vi "Get Connection Settings.vi"(11 "Model in":refnum<class "Model.lvclass">) -> (2 "Connection Settings":T1={"Pressure Servo Valve 1 DAC"=1, "Pressure Servo Valve 2 DAC"=2, "Turbo Valve DAC"=3, "Load Cell ADC"=1, "FC1 ILC Port"="", "FC2 ILC Port"="", "Tovey A-B Port"="", "Tovey C-F Port"="", "Tovey D-E Port"="", "FC1 ILC Protocol"=enum."RS485", "FC2 ILC Protocol"=enum."RS485", "Tovey A-B Protocol"=enum."RS485", "Tovey C-F Protocol"=enum."RS485", "Tovey D-E Protocol"=enum."RS485", "Tovey A-B Address"=3, "Tovey C-F Address"=1, "Tovey D-E Address"=1, "Bias DAC"=4, "Axial Push Channel"="ai0", "Axial Pull Channel"="ai1", "Lateral Push Channel"="ai2", "Lateral Pull Channel"="ai3", "TV Control"="ao0", "TV Bias"="ao1", "Rate"=200} {"Rate" min=1; "Bias DAC" min=1 max=4; "Tovey D-E Address" min=1; "Tovey C-F Address" min=1; "Tovey A-B Address" min=1; "Load Cell ADC" min=1 max=4; "Turbo Valve DAC" min=1 max=4; "Pressure Servo Valve 2 DAC" min=1 max=4; "Pressure Servo Valve 1 DAC" min=1 max=4}, 3 "Model out":refnum<class "Model.lvclass">)   [LabVIEW 2015, in "Model.lvclass"]
uses:
  Model.lvclass
  Typedefs/Connection Settings.ctl
  <userlib>/Common/SerialProtocols/Configuration/SerialProtocol.ctl
  Model.lvclass/Model.ctl
  <userlib>/Common/SerialProtocols/SerialProtocols.lvlib
  Typedefs/FAMT Typedefs.lvlib
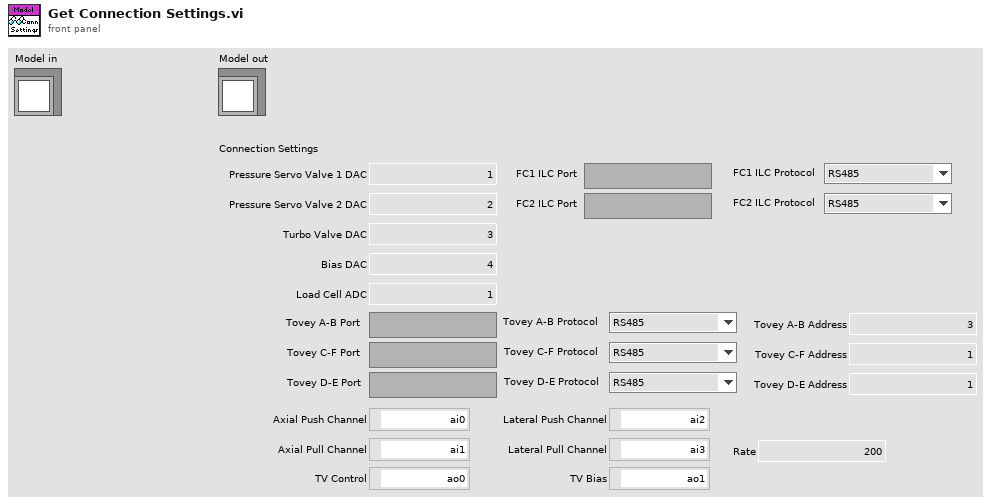
[diagram p1: front panel]
types:
  T1 = typedef "FAMT Typedefs.lvlib/Connection Settings.ctl" = cluster{"Pressure Servo Valve 1 DAC":u8, "Pressure Servo Valve 2 DAC":u8, "Turbo Valve DAC":u8, "Load Cell ADC":u8, "FC1 ILC Port":refnum<visa-resource-name>, "FC2 ILC Port":refnum<visa-resource-name>, "Tovey A-B Port":refnum<visa-resource-name>, "Tovey C-F Port":refnum<visa-resource-name>, "Tovey D-E Port":refnum<visa-resource-name>, "FC1 ILC Protocol":T2, "FC2 ILC Protocol":T2, "Tovey A-B Protocol":T2, "Tovey C-F Protocol":T2, "Tovey D-E Protocol":T2, "Tovey A-B Address":u8, "Tovey C-F Address":u8, "Tovey D-E Address":u8, "Bias DAC":u8, "Axial Push Channel":refnum<k21>, "Axial Pull Channel":refnum<k21>, "Lateral Push Channel":refnum<k21>, "Lateral Pull Channel":refnum<k21>, "TV Control":refnum<k21>, "TV Bias":refnum<k21>, "Rate":u8}
  T2 = typedef "SerialProtocols.lvlib/SerialProtocol.ctl" = enum16{"RS232", "RS485", "SerialSimulator"}
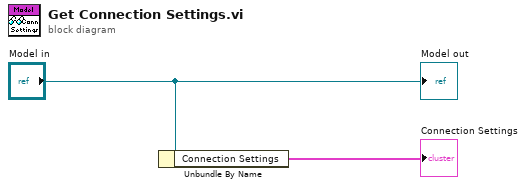
[diagram p0: block diagram]
diagram:
  n1 = Unbundle By Name("Model in") -> ("Connection Settings"=→"Connection Settings":T1)
  "Model out" <- "Model in"
